vi "Detect Frequency.vi"() -> ()   [LabVIEW 2012]
uses:
  <vilib>/DAQmx/read.llb/DAQmx Read (Analog Wfm 1Chan NSamp).vi
  <vilib>/DAQmx/create/channels.llb/DAQmx Create Channel (AI-Voltage-Basic).vi
  <vilib>/DAQmx/configure/timing.llb/DAQmx Timing (Sample Clock).vi
  <vilib>/measure/matone.llb/Extract Single Tone Information 1 Chan.vi
  <vilib>/DAQmx/miscellaneous.llb/DAQmx Fill In Error Info.vi
  <resource>/objmgr/daqmx.rc
  <vilib>/measure/NI_MAPro.lvlib
panel:
  out "Detected Frequency":dbl
  in  "Stop":bool
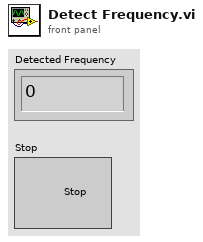
[diagram p1: front panel]
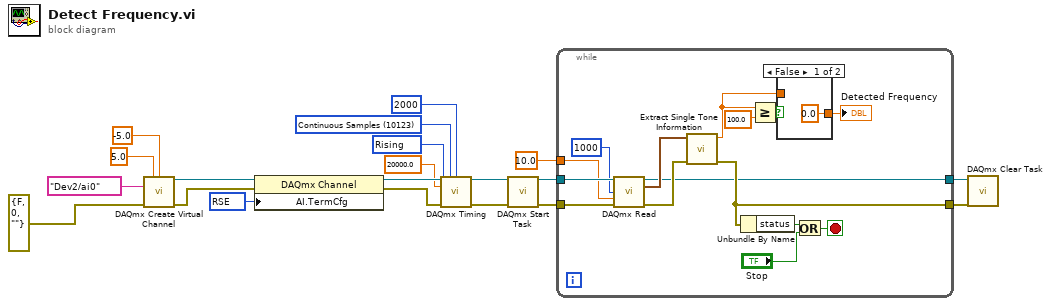
[diagram p0: block diagram]
diagram:
  w6 = 10280 items=["Rising"=10280, "Falling"=10171] ("active edge")
  w9 = 10123 items=["Finite Samples"=10178, "Continuous Samples"=10123, "Hardware Timed Single Point"=12522] ("sample mode")
  w10 = 10083 items=["RSE"=10083, "NRSE"=10078, "Differential"=10106, "Pseudodifferential"=12529] ("AI.TermCfg")
  n1 = call-poly <vilib>:"DAQmx Create Virtual Channel.vi"("maximum value"=5.0, "minimum value"=-5.0, "physical channels"=tag "Dev2/ai0", "error in"=errorcluster {"status"=FALSE, "code"=0, "source"=""} ("error constant")) -> ("task out"=w15:refnum<k21>, "error out"=w16:errorcluster)  [unwired: 10 in]
  n2 = property class="DAQmx Channel"(reference=w15, error in=w16, "AI.TermCfg"=w10) -> (reference out=w17:refnum<k21>, error out=w18:errorcluster)
  n3 = call-poly <vilib>:"DAQmx Timing.vi"("task/channels in"=w17, "sample mode"=w9, "samples per channel"=2000, "rate"=20000.0, "active edge"=w6, "error in"=w18) -> ("task out"=w20:refnum<k21>, "error out"=w19:errorcluster)  [unwired: 8 in]
  n4 = call <vilib>:"DAQmx Start Task.vi"("task/channels in"=w20, "error in"=w19) -> ("task out"=w4:refnum<k21>, "error out"=w5:errorcluster)  [unwired: 12 in]
  n5 = while {
    tunnel: w5 -> [w35]
    tunnel: w4 -> [w34]
    tunnel: 10.0 ("rate") -> [w33]
    tunnel: [w29] -> w2
    tunnel: [w31] -> w1
    stop <- w27 stop-if-true
    n6 = call-poly <vilib>:"DAQmx Read.vi"("task/channels in"=w34, "number of samples per channel"=1000, "timeout"=w33, "error in"=w35) -> ("task out"=w29:refnum<k21>, "data"=w30:waveform(dbl), "error out"=w32:errorcluster)  [unwired: 9 in]
    n7 = call-poly <vilib>:"Extract Single Tone Information.vi"("error in (no error)"=w32, "time signal in"=w30) -> ("error out"=w31:errorcluster, "detected frequency"=w22:dbl)  [unwired: 4 in, 4 out]
    n8 = Unbundle By Name(w31) -> ("status"=w28:bool)
    n9 = Greater Or Equal?(x=w22, y=100.0) -> (x >= y?=w24:bool)
    n10 = case shown="False" w24 {
      tunnel: w22 -> [_ w37]
      tunnel: [0.0 ("detected frequency") w37] -> w21
      frame False {
      }
      frame True {
      }
    }
    "Detected Frequency" <- w21
    n11 = Or(x=w28, y="Stop") -> (x .or. y?=w27:bool)
  }
  n12 = call <vilib>:"DAQmx Clear Task.vi"("task in"=w2, "error in"=w1) -> ()  [unwired: 13 in, 1 out]
